vi "(Var)RedNoah3 Info.vi"() -> ()   [LabVIEW 2020]
uses:
  Controls/(Ctrl)Launcher_RedNoah3 Edition.ctl
panel:
  in  "RedNoah3 Edition":T1
  in  "RedNoah3 SN":string
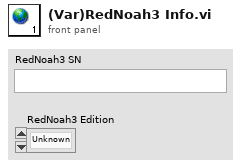
[diagram p1: front panel]
types:
  T1 = typedef "(Ctrl)Launcher_RedNoah3 Edition.ctl" = enum16{"Unknown", "Single Board", "Sensor Package"}
diagram:
